vi "V50 Report Range (SubVI).vi"(0 "NI_report in":refnum<class "NI_report.lvclass">, 5 "SampleID":string, 11 "error in (no error)":errorcluster) -> (4 "NI_report out":refnum<class "NI_report.lvclass">, 15 "error out":errorcluster)   [LabVIEW 2015]
uses:
  <vilib>/Utility/NIReport.llb/NI_report.lvclass
panel:
  out "appended array":string[][](array[string])
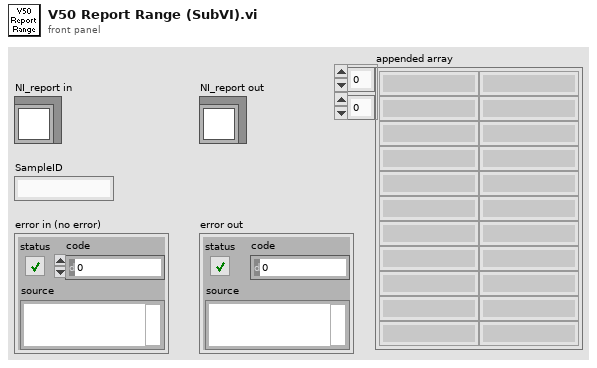
[diagram p1: front panel]
types:
  T1 = cluster{"position (excel)":cluster{"row":i32, "column":i32}, "name (excel)":string, "bookmark (word)":string}
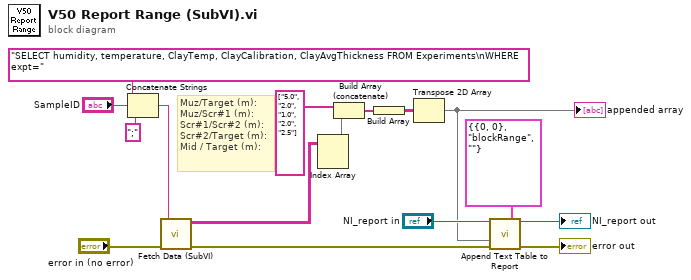
[diagram p0: block diagram]
diagram:
  # "Muz/Target (m):\nMuz/Scr#1 (m):\nScr#1/Scr#2 (m):\nScr#2/Target (m):\nMid / Target (m):"
  n1 = Concatenate Strings("SELECT humidity, temperature, ClayTemp, ClayCalibration, ClayAvgThickness FROM Experiments\nWHERE expt=" ("query string"), "SampleID", ";" ("string")) -> (w13:string)
  n2 = call "Fetch Data (SubVI).vi"("error IN"="error in (no error)", "query string"=w13) -> ("error OUT"=w7:errorcluster, "recordset data"=w5:string[][])  [unwired: 4 out]
  n3 = Index Array(array=w5) -> (element=w4:string[])  [unwired: 2 in]
  n4 = Build Array (concatenate)(string[] ["5.0", "2.0", "1.0", "2.0", "2.5"] ("new element/subarray"), w4) -> (w6:string[])
  n5 = Build Array(w6) -> (w2:string[][])
  n6 = Transpose 2D Array(2D array=w2) -> (transposed array=w1:string[][])
  "appended array" <- w1
  n7 = call-dynamic "Append Text Table to Report.vi"("report in"="NI_report in", "MS Office parameters"=T1 {"position (excel)"={"row"=0, "column"=0}, "name (excel)"="blockRange", "bookmark (word)"=""}, "text data"=w1, "error in (no error)"=w7) -> ("report out"=→"NI_report out":refnum<class "NI_report.lvclass">, "error out"=→"error out":errorcluster)  [unwired: 8 in, 2 out]
